vi "simple element vs typedef.vi"(11 "elements":variant[](array[variant])) -> (3 "simple identifiers":string[](array[string]))   [LabVIEW 2026]
uses:
  <vilib>/Utility/Data Type/NI_Data Type.lvlib
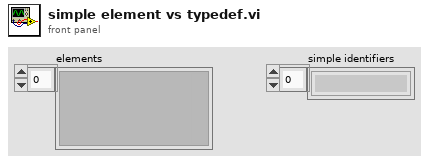
[diagram p1: front panel]
types:
  T1 = typedef "NI_Data Type.lvlib/Data Type.ctl" = enum8{"Invalid Type", "Void", "I8", "I16", "I32", "I64", "U8", "U16", "U32", "U64", "Single Float", "Double Float", "Extended Float", "Single Complex", "Double Complex", "Extended Complex", "Enum U8", "Enum U16", "Enum U32", "Enum U64", "Single Float With Unit", "Double Float With Unit", "Extended Float With Unit", "Single Complex with Unit", "Double Complex with Unit", "Extended Complex with Unit", "Boolean", "String", "Path", "Picture", "Tag", "Array", "Cluster", "Variant", "LV Variant", "Waveform", "Timestamp", "Digital Waveform", "Digital Data", "ExpressData", "Refnum", "External Data", "VI", "Poly VI", "LabVIEW Class Instance", "Fixed Point", "Set Collection", "Map Collection"}
  T2 = typedef "NI_Data Type.lvlib/Type Definition Info.ctl" = cluster{"Name":string, "Timestamp":u32}
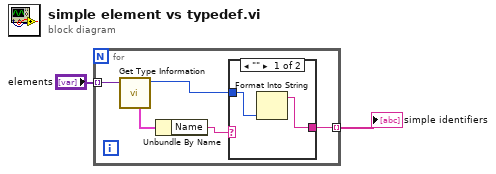
[diagram p0: block diagram]
diagram:
  n1 = for {
    tunnel: "elements" -> [w7] mode=indexing
    tunnel: [w4] -> w2 mode=indexing
    n2 = call <vilib>:"Get Type Information.vi"("variant"=w7) -> ("type"=w3:T1, "type definition info"=w6:T2)  [unwired: 6 in, 3 out]
    n3 = Unbundle By Name(w6) -> ("Name"=w5:string)
    n4 = case shown="\"\"" w5 {
      selector: w5 -> [_ w10]
      tunnel: [w8 w10] -> w4
      tunnel: w3 -> [w9 _]
      frame "" {
        n5 = Format Into String(w9) -> (resulting string=w8:string)  [unwired: 3 in, 1 out]
      }
      frame Default {
      }
    }
  }
  "simple identifiers" <- w2
